vi "GUI - WaveFile (V2.00).vi"(0 "Time Data IN":refnum<class "GSwFormDSP.lvclass">, 5 "error in (no error)":errorcluster, 6 "Scale Factor":dbl=1.0 min=0.999993656453662 format="%#.2g", 7 "Application Name":string="GSwForm", 8 "Filename Option (Write)":T2(ring), 9 "State Queue":string[](array[string])=["SC >>> Initialize"], 11 "Wave - READ":path, 13 "Wave - WRITE":path) -> (14 "SubVI Time Data DUP":refnum<class "GSwFormDSP.lvclass">, 19 "error out":errorcluster)   [LabVIEW 2022 SP3, in "WaveFile.lvclass"]
uses:
  WaveFile.lvclass
  API/GSwFormDSP_class/GSwFormDSP.lvclass
  protected/Multi Signals Save Option.ctl
  <vilib>/Utility/sysdir.llb/System Directory Type.ctl
  W:/projects/archives/23 Charette AI Group/SPWB/API/Generic Utilities_class/Generic Utilities.lvclass
  API/Generic Utilities_class/Generic Utilities.lvclass
  <vilib>/addons/_AddQ/G#Object/G#Object.lvclass
panel:
  in  "Task":T1(tab)
  in  "READ - Multiple Files":path[](array[path])
  out "Time Data - READ":waveform(dbl)[](graph)
  in  "READ - Select Wave File":bool
  in  "READ - Select Multiple Wave File":bool
  in  "Multi Signal Save Option":T3
  out "Signal Name Tag":string="{ Signal Name }"
  in  "Open New TDF window":bool caption="Open the new Wave File in a New TDF window"
  in  "Suffix":string
  in  "Extension":string=".wav"
  in  "Fade IN and OUT":bool
  in  "Force Fs=44100Hz":bool
  in  "Filename":string
  in  "Unit Option":enum16{"No Change", "dB (Ref 20e-6 EU)"}(ring)
  in  "Unit":string
  in  "Save (GUI)":bool
  out "State History":string[](array[string])
  out "State Index":i32
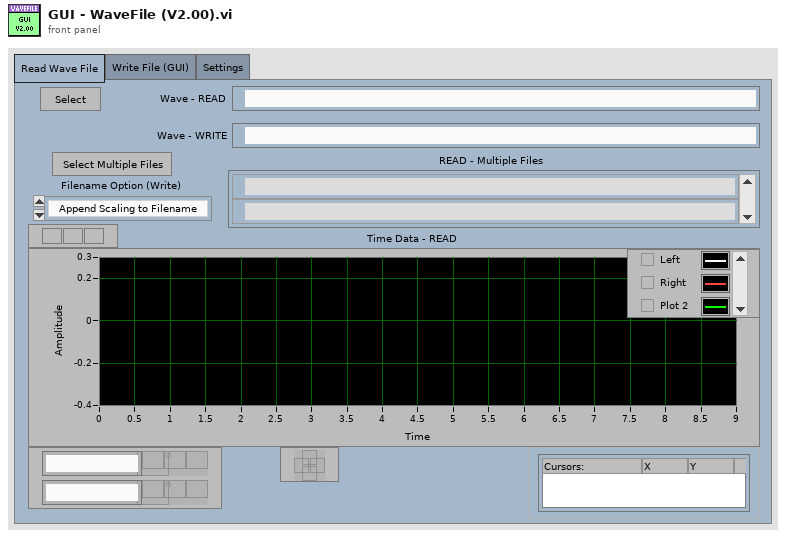
[diagram p1: front panel]
types:
  T1 = enum32{"Read Wave File", "Write File (GUI)", "Settings"}
  T2 = enum16{"Append Scaling to Filename", "No Scaling Info"}
  T3 = typedef "WaveFile.lvclass/Multi Signals Save Option.ctl" = enum16{"One wave file per signal", "Concatenate ALL signals to a single file", "Stereo (Ch1 is Left, Ch2 is Right)", "Stereo (Ch1 is Right, Ch2 is Left)"}
  T4 = enum8{"Enabled", "Disabled", "Disabled and Grayed Out"}
  T5 = enum32{"Invalid", "Standard", "Closed", "Hidden", "Minimized", "Maximized"}
  T6 = enum32{"Invalid", "Default", "Floating", "Floating/Auto-Hide", "Modal"}
  T7 = typedef "System Directory Type.ctl" = i32
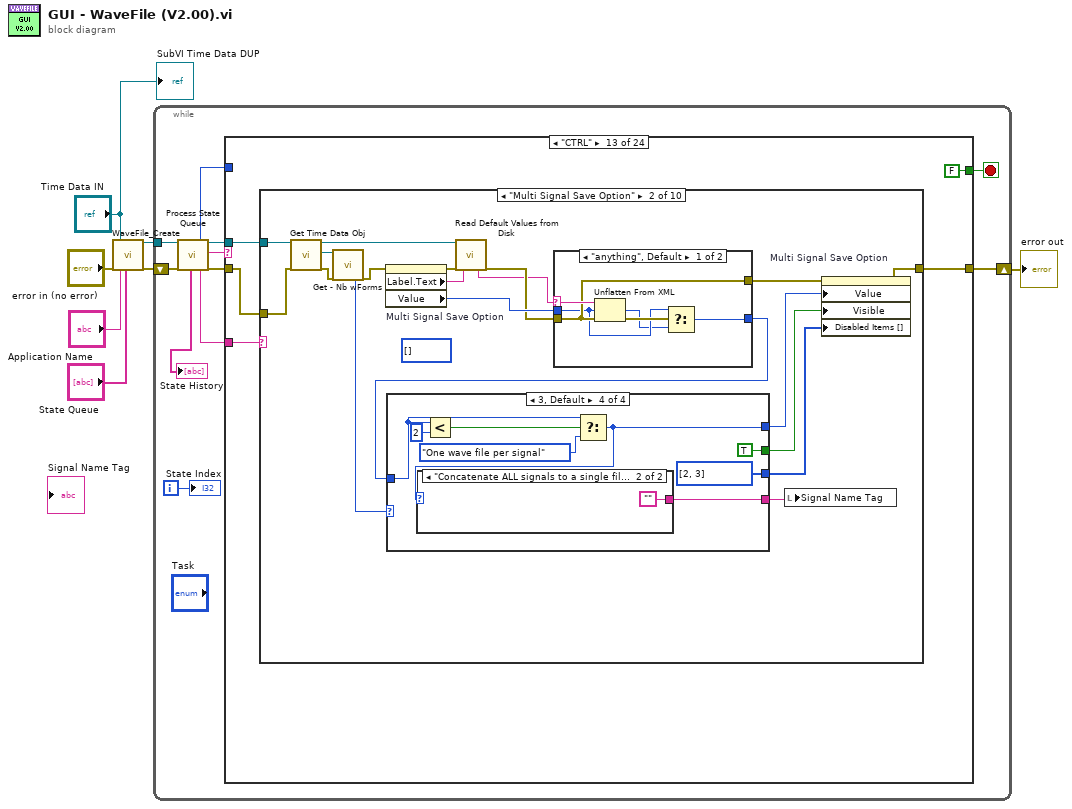
[diagram p0: block diagram]
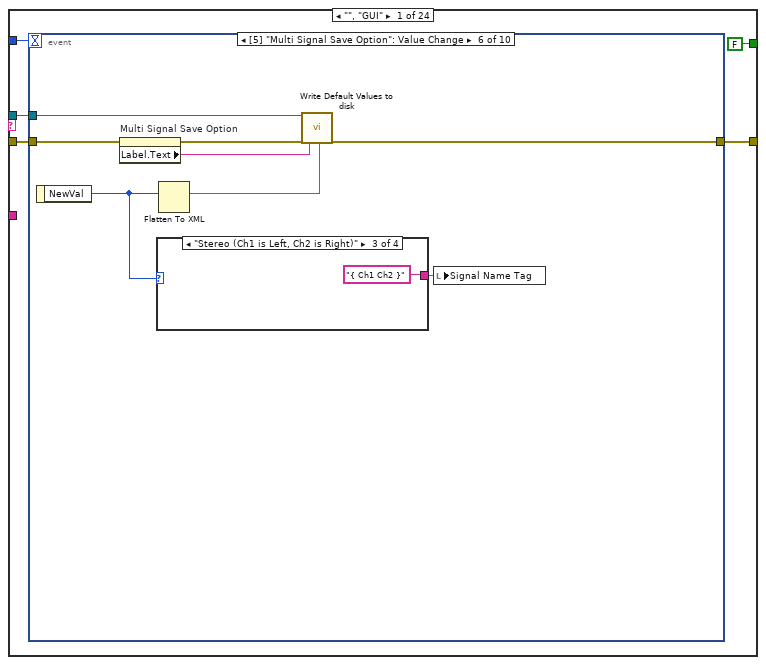
[diagram p2: hidden frame]
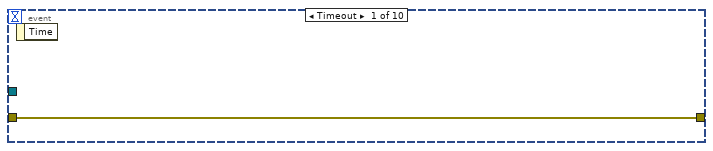
[diagram p3: hidden frame]
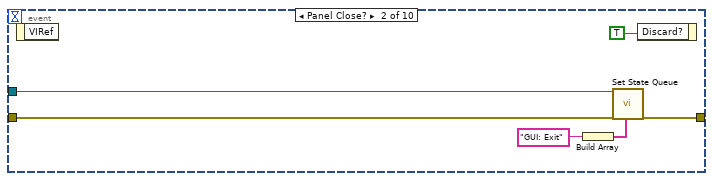
[diagram p4: hidden frame]
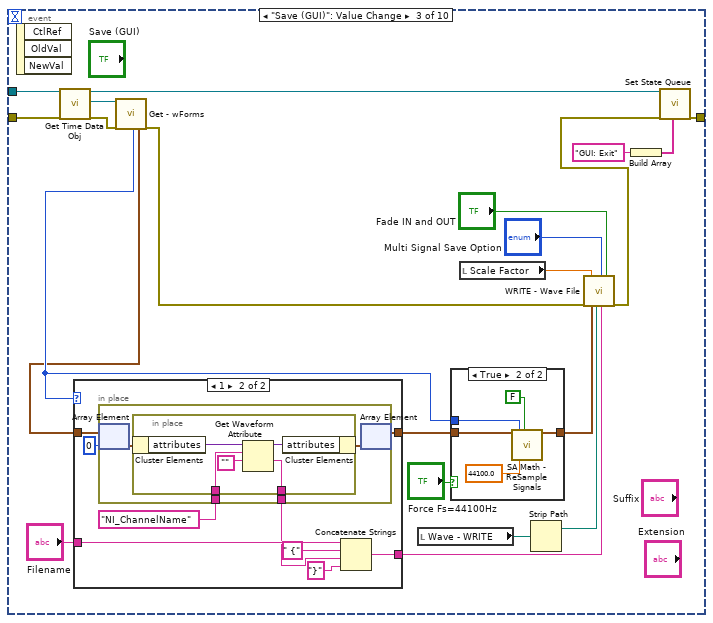
[diagram p5: hidden frame]
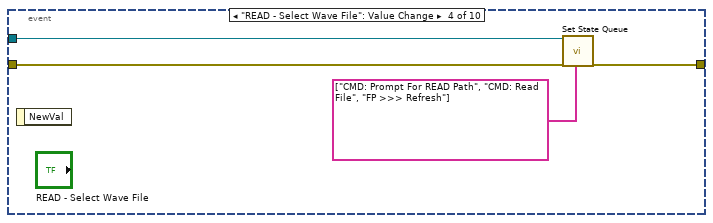
[diagram p8: hidden frame]
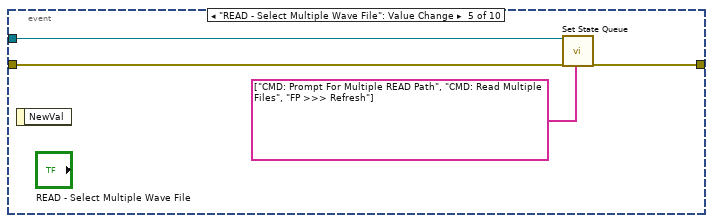
[diagram p9: hidden frame]
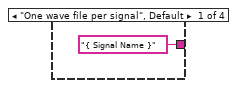
[diagram p10: hidden frame]
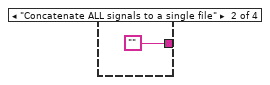
[diagram p11: hidden frame]
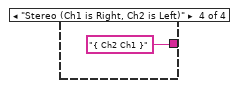
[diagram p12: hidden frame]
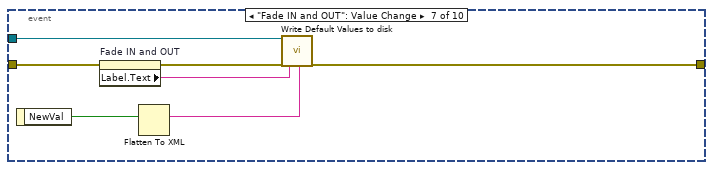
[diagram p13: hidden frame]
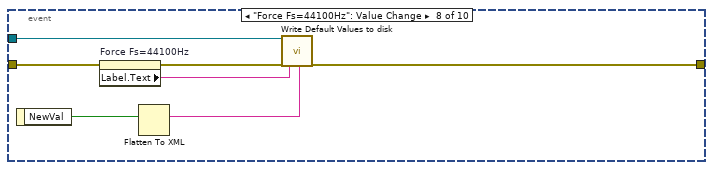
[diagram p14: hidden frame]
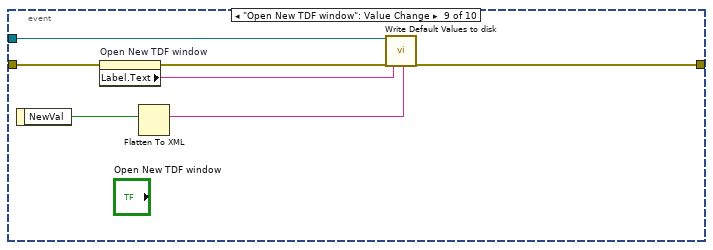
[diagram p15: hidden frame]
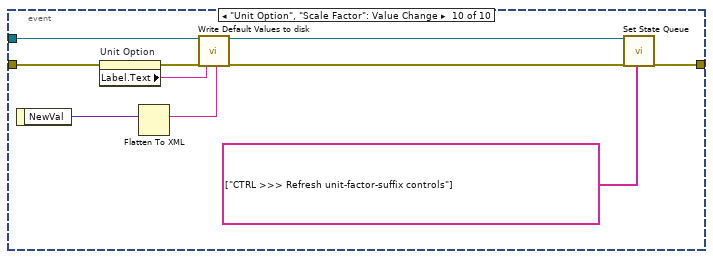
[diagram p16: hidden frame]
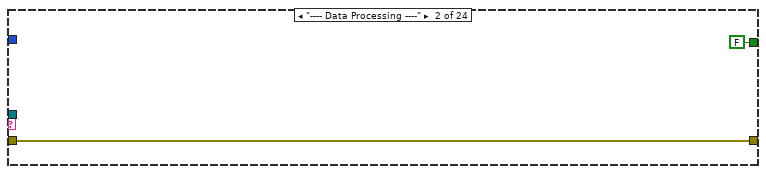
[diagram p17: hidden frame]
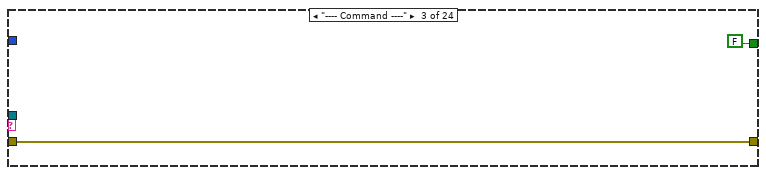
[diagram p18: hidden frame]
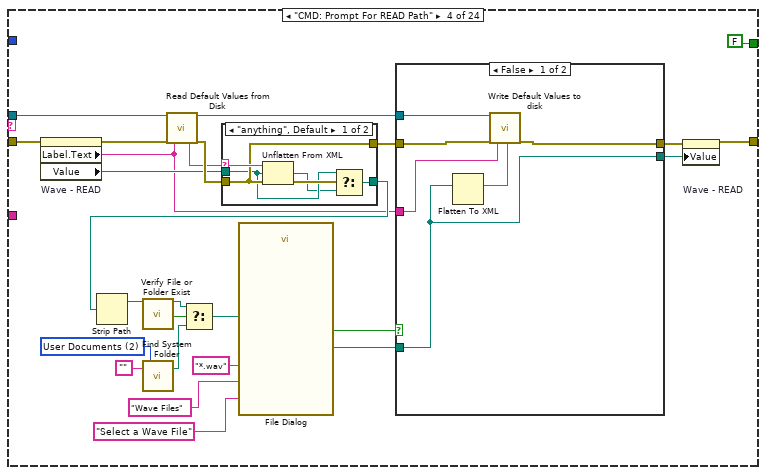
[diagram p19: hidden frame]
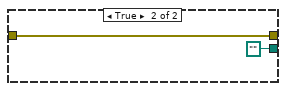
[diagram p20: hidden frame]
diagram:
  n1 = call "WaveFile_Create.vi"("error in (no error)"="error in (no error)", "Time Data"="Time Data IN", "Application Name"="Application Name", "State Queue"="State Queue") -> ("reference out"=w7:refnum<class "WaveFile.lvclass">, "error out"=w6:errorcluster)  [unwired: 14 in]
  n2 = while {
    shift-right: [w9] -> w2
    shift-left: w6 -> [w15]
    tunnel: w7 -> [w16]
    i -> [w17]
    stop <- w18 stop-if-true
    n3 = call "Process State Queue.vi"("reference in"=w16, "error in (no error)"=w15) -> ("State History"=→"State History":string[], "Timeout"=w14:i32, "State Option"=w11:string, "reference out"=w13:refnum<class "WaveFile.lvclass">, "Current State"=w12:string, "error out"=w10:errorcluster)  [unwired: 10 in, 2 out]
    n4 = case shown="\"CTRL\"" w12 {
      selector: w12 -> [_ _ _ _ _ _ _ _ _ _ _ _ _ _ _ _ _ _ _ _ w668 _ _ _]
      tunnel: w13 -> [w21 _ _ w158 w201 w243 w269 w280 w288 _ w316 _ w324 w530 _ w571 w594 w625 w650 _ _ _ _ w677]
      tunnel: [FALSE FALSE FALSE FALSE FALSE FALSE FALSE FALSE FALSE FALSE FALSE FALSE FALSE FALSE FALSE FALSE TRUE FALSE FALSE FALSE FALSE FALSE FALSE TRUE] -> w18
      tunnel: w14 -> [w22 _ _ _ _ _ _ _ _ _ _ _ _ _ _ _ _ _ _ _ _ _ _ _]
      tunnel: w11 -> [_ _ _ _ _ _ _ _ _ _ w312 _ w325 w527 _ w564 _ w634 _ _ _ _ _ _]
      tunnel: w10 -> [w20 w130 w132 w157 w200 w242 w268 w279 w290 w310 w315 w320 w322 w529 w554 w568 w591 w624 w651 w664 w666 w671 w674 w676]
      tunnel: [w19 w130 w132 w141 w185 w226 w267 w278 w289 w310 w314 w320 w323 w528 w554 w556 w590 w622 w647 w664 w666 errorcluster {"status"=FALSE, "code"=0, "source"=""} ("error out") w674 w678] -> w9
      frame "", "GUI" {
        n5 = event shown="[5] \"Multi Signal Save Option\": Value Change" {
          selector: _ -> [_ _ _ _ _ _ _ _ _ _]
          dyn-events: _ -> [_ _ _ _ _ _ _ _ _ _]
          timeout: w22 -> [_ _ _ _ _ _ _ _ _ _]
          tunnel: w21 -> [_ w28 w49 w81 w85 w93 w104 w111 w118 w128]
          tunnel: w20 -> [w24 w27 w48 w80 w84 w94 w105 w112 w119 w129]
          tunnel: [w24 w26 w50 w82 w86 w89 w99 w106 w113 w121] -> w19
          event Timeout {
            n6 = event-data() -> ()  [unwired: 1 in, 1 out]
          }
          event Panel Close? {
            n7 = event-data() -> ()  [unwired: 1 in, 1 out]
            n8 = Build Array("GUI: Exit") -> (w25:string[])
            n9 = call "Set State Queue.vi"("reference in"=w28, "error in (no error)"=w27, "State Queue"=w25) -> ("error out"=w26:errorcluster)  [unwired: 15 in, 1 out]
            n10 = event-data("Discard?"=TRUE) -> ()  [unwired: 1 in, 1 out]
          }
          event "Save (GUI)": Value Change {
            n11 = event-data() -> ()  [unwired: 1 in, 3 out]
            n12 = call "Get Time Data Obj.vi"("reference in"=w49, "error in (no error)"=w48) -> ("reference out"=w45:refnum<class "WaveFile.lvclass">, "Time data ref"=w47:refnum<class "GSwFormDSP.lvclass">, "error out"=w46:errorcluster)  [unwired: 15 in]
            n13 = call-dynamic "Get - wForms.vi"("reference in"=w47, "error in (no error)"=w46) -> ("Nb Signals"=w34:i32, "wForms"=w33:waveform(dbl)[], "error out"=w41:errorcluster)  [unwired: 14 in, 1 out]
            n14 = case shown="1" w34 {
              tunnel: [w54 w57] -> w38
              tunnel: "Filename" -> [w54 w60]
              tunnel: [w53 w62] -> w37
              tunnel: w33 -> [w53 w63]
              frame 0, Default {
              }
              frame 1 {
                n15 = in-place {
                  in-place-border: "NI_ChannelName" ("Att - wform Name") -> [w65]
                  in-place-border: [w64] -> w58
                  n16 = in-place-array #1(w63, 0) -> (w67:waveform(dbl))
                  n17 = in-place {
                    in-place-border: w65 -> [w70]
                    in-place-border: [w68] -> w64
                    n18 = in-place-cluster #2(w67) -> ("attributes"=w72:variant)
                    n19 = Get Waveform Attribute(5:"", 6:w70, 7:w72) -> (1:w68:string, 3:w71:variant)  [unwired: 1 in, 2 out]
                    n20 = in-place-cluster #2("attributes"=w71) -> (w66:waveform(dbl))
                  }
                  n21 = in-place-array #1(w66) -> (w62:waveform(dbl)[])  [unwired: 1 out]
                }
                n22 = Concatenate Strings(w60, " {" ("string"), w58, "}" ("string")) -> (w57:string)
              }
            }
            n23 = local read "Wave - WRITE"() -> (w42:path)
            n24 = case shown="True" "Force Fs=44100Hz" {
              tunnel: [w73 w77] -> w43
              tunnel: w37 -> [w73 w78]
              tunnel: w34 -> [_ w74]
              frame False {
              }
              frame True {
                n25 = call "SA Math - ReSample Signals.vi"("Time in"=w78, "Nb Signals"=w74, "New Fs"=44100.0, "Anotate Signal Name"=FALSE) -> ("Time out"=w77:waveform(dbl)[])  [unwired: 14 in, 1 out]
              }
            }
            n26 = local read "Scale Factor"() -> (w35:dbl)
            n27 = Strip Path(path=w42) -> (stripped path=w40:path)  [unwired: 1 out]
            n28 = call "WRITE - Wave File.vi"("error in (no error)"=w41, "Scaling Factor"=w35, "wForms"=w43, "Path"=w40, "Multi Signal Save Option"="Multi Signal Save Option", "Filename"=w38, "Fade IN and OUT"="Fade IN and OUT") -> ("error out"=w36:errorcluster)  [unwired: 12 in]
            n29 = Build Array("GUI: Exit") -> (w51:string[])
            n30 = call "Set State Queue.vi"("reference in"=w45, "error in (no error)"=w36, "State Queue"=w51) -> ("error out"=w50:errorcluster)  [unwired: 15 in, 1 out]
          }
          event "READ - Select Wave File": Value Change {
            n31 = event-data() -> ()  [unwired: 1 in, 1 out]
            n32 = call "Set State Queue.vi"("reference in"=w81, "error in (no error)"=w80, "State Queue"=string[] ["CMD: Prompt For READ Path", "CMD: Read File", "FP >>> Refresh"]) -> ("error out"=w82:errorcluster)  [unwired: 15 in, 1 out]
          }
          event "READ - Select Multiple Wave File": Value Change {
            n33 = event-data() -> ()  [unwired: 1 in, 1 out]
            n34 = call "Set State Queue.vi"("reference in"=w85, "error in (no error)"=w84, "State Queue"=string[] ["CMD: Prompt For Multiple READ Path", "CMD: Read Multiple Files", "FP >>> Refresh"]) -> ("error out"=w86:errorcluster)  [unwired: 15 in, 1 out]
          }
          event Value Change {
            n35 = event-data() -> ("NewVal"=w88:T3)  [unwired: 1 in]
            n36 = property on="Multi Signal Save Option" class="Enum (strict)"(error in=w94) -> (error out=w92:errorcluster, "Label.Text"=w91:string)  [unwired: 1 in, 1 out]
            n37 = case shown="\"Stereo (Ch1 is Left, Ch2 is Right)\"" w88 {
              tunnel: ["{ Signal Name }" "" "{ Ch1 Ch2 }" "{ Ch2 Ch1 }"] -> w87
              frame "One wave file per signal", Default {
              }
              frame "Concatenate ALL signals to a single file" {
              }
              frame "Stereo (Ch1 is Left, Ch2 is Right)" {
              }
              frame "Stereo (Ch1 is Right, Ch2 is Left)" {
              }
            }
            n38 = Flatten To XML(6:w88) -> (2:w90:string)
            n39 = call-dynamic "Write Default Values to disk.vi"("reference in"=w93, "error in (no error)"=w92, "Control Label"=w91, "Value (XML String)"=w90) -> ("error out"=w89:errorcluster)  [unwired: 14 in, 1 out]
            n40 = local write "Signal Name Tag"(w87) -> ()
          }
          event "Fade IN and OUT": Value Change {
            n41 = event-data() -> ("NewVal"=w101:bool)  [unwired: 1 in]
            n42 = property on="Fade IN and OUT" class="Bool (strict)"(error in=w105) -> (error out=w103:errorcluster, "Label.Text"=w102:string)  [unwired: 1 in, 1 out]
            n43 = Flatten To XML(6:w101) -> (2:w100:string)
            n44 = call-dynamic "Write Default Values to disk.vi"("reference in"=w104, "error in (no error)"=w103, "Control Label"=w102, "Value (XML String)"=w100) -> ("error out"=w99:errorcluster)  [unwired: 14 in, 1 out]
          }
          event "Force Fs=44100Hz": Value Change {
            n45 = event-data() -> ("NewVal"=w108:bool)  [unwired: 1 in]
            n46 = property on="Force Fs=44100Hz" class="Bool (strict)"(error in=w112) -> (error out=w110:errorcluster, "Label.Text"=w109:string)  [unwired: 1 in, 1 out]
            n47 = Flatten To XML(6:w108) -> (2:w107:string)
            n48 = call-dynamic "Write Default Values to disk.vi"("reference in"=w111, "error in (no error)"=w110, "Control Label"=w109, "Value (XML String)"=w107) -> ("error out"=w106:errorcluster)  [unwired: 14 in, 1 out]
          }
          event "Open New TDF window": Value Change {
            n49 = event-data() -> ("NewVal"=w115:bool)  [unwired: 1 in]
            n50 = property on="Open New TDF window" class="Bool (strict)"(error in=w119) -> (error out=w117:errorcluster, "Label.Text"=w116:string)  [unwired: 1 in, 1 out]
            n51 = Flatten To XML(6:w115) -> (2:w114:string)
            n52 = call-dynamic "Write Default Values to disk.vi"("reference in"=w118, "error in (no error)"=w117, "Control Label"=w116, "Value (XML String)"=w114) -> ("error out"=w113:errorcluster)  [unwired: 14 in, 1 out]
          }
          event "Unit Option", "Scale Factor": Value Change {
            n53 = event-data() -> ("NewVal"=w125:variant)  [unwired: 1 in]
            n54 = property on="Unit Option" class="Enum (strict)"(error in=w129) -> (error out=w127:errorcluster, "Label.Text"=w126:string)  [unwired: 1 in, 1 out]
            n55 = Flatten To XML(6:w125) -> (2:w124:string)
            n56 = call-dynamic "Write Default Values to disk.vi"("reference in"=w128, "error in (no error)"=w127, "Control Label"=w126, "Value (XML String)"=w124) -> ("reference out"=w120:refnum<class "WaveFile.lvclass">, "error out"=w122:errorcluster)  [unwired: 14 in]
            n57 = call "Set State Queue.vi"("reference in"=w120, "error in (no error)"=w122, "State Queue"=string[] ["CTRL >>> Refresh unit-factor-suffix controls"]) -> ("error out"=w121:errorcluster)  [unwired: 15 in, 1 out]
          }
        }
      }
      frame "---- Data Processing ----" {
      }
      frame "---- Command ----" {
      }
      frame "CMD: Prompt For READ Path" {
        w148 = T7 2 items=["User Home"=0, "User Desktop"=1, "User Documents"=2, "User Application Data"=3, "User Preferences"=4, "User Temporary"=5, "Public Documents"=6, "Public Application Data"=7, "Public Preferences"=8, "Public Cache"=13, "System Core Libraries"=9, "System Installed Libraries"=10, "Application Files"=11, "Boot Volume Root"=12] ("system directory type")
        n58 = property on="Wave - READ" class="Path"(error in=w157) -> (error out=w156:errorcluster, "Label.Text"=w136:string, "Value"=w154:path)  [unwired: 1 in, 1 out]
        n59 = call "Find System Folder.vi"("Application Name"="", "system directory type"=w148) -> ("System Folder"=w147:path)  [unwired: 16 in, 1 out]
        n60 = call-dynamic "Read Default Values from Disk.vi"("reference in"=w158, "error in (no error)"=w156, "Control Label"=w136) -> ("Value (XML String)"=w134:string, "reference out"=w137:refnum<class "WaveFile.lvclass">, "error out"=w155:errorcluster)  [unwired: 14 in]
        n61 = case shown="\"anything\", Default" w134 {
          selector: w134 -> [w173 _]
          tunnel: [w168 w175] -> w153
          tunnel: w154 -> [w170 w175]
          tunnel: w155 -> [w171 w174]
          tunnel: [w171 w174] -> w139
          frame "anything", Default {
            n62 = Unflatten From XML(xml string=w173, type=w170, error in (no error)=w171) -> (value=w169:path, error out=w172:errorcluster)
            n63 = Select(t=w170, s=w172, f=w169) -> (s? t:f=w168:path)
          }
          frame "" {
            # "Either the file was not found or there was some error"
          }
        }
        n64 = Strip Path(path=w153) -> (stripped path=w152:path)  [unwired: 1 out]
        n65 = call "Verify File or Folder Exist.vi"("path"=w152) -> ("dup path"=w150:path, "file or folder exists?"=w151:bool)  [unwired: 16 in, 1 out]
        n66 = Select(t=w150, s=w151, f=w147) -> (s? t:f=w149:path)
        n67 = call "File Dialog"("start path"=w149, "button label"="Select a Wave File", "pattern (all files)"="*.wav", "pattern label"="Wave Files") -> ("selected path"=w135:path, "cancelled"=w142:bool)  [unwired: 8 in, 2 out]
        n68 = case shown="False" w142 {
          tunnel: [w161 w167] -> w140
          tunnel: w139 -> [w162 w167]
          tunnel: [w160 path ""] -> w138
          tunnel: w137 -> [w164 _]
          tunnel: w136 -> [w163 _]
          tunnel: w135 -> [w160 _]
          frame False {
            n69 = Flatten To XML(6:w160) -> (2:w165:string)
            n70 = call-dynamic "Write Default Values to disk.vi"("reference in"=w164, "error in (no error)"=w162, "Control Label"=w163, "Value (XML String)"=w165) -> ("error out"=w161:errorcluster)  [unwired: 14 in, 1 out]
          }
          frame True {
          }
        }
        n71 = property on="Wave - READ" class="Path"(error in=w140, "Value"=w138) -> (error out=w141:errorcluster)  [unwired: 1 in, 1 out]
      }
      frame "CMD: Prompt For Multiple READ Path" {
        w192 = T7 2 items=["User Home"=0, "User Desktop"=1, "User Documents"=2, "User Application Data"=3, "User Preferences"=4, "User Temporary"=5, "Public Documents"=6, "Public Application Data"=7, "Public Preferences"=8, "Public Cache"=13, "System Core Libraries"=9, "System Installed Libraries"=10, "Application Files"=11, "Boot Volume Root"=12] ("system directory type")
        n72 = property on="READ - Multiple Files" class="Arr (strict)"(error in=w200) -> (error out=w199:errorcluster, "Label.Text"=w180:string, "Value"=w197:path[])  [unwired: 1 in, 1 out]
        n73 = call "Find System Folder.vi"("Application Name"="", "system directory type"=w192) -> ("System Folder"=w191:path)  [unwired: 16 in, 1 out]
        n74 = call-dynamic "Read Default Values from Disk.vi"("reference in"=w201, "error in (no error)"=w199, "Control Label"=w180) -> ("Value (XML String)"=w176:string, "reference out"=w181:refnum<class "WaveFile.lvclass">, "error out"=w198:errorcluster)  [unwired: 14 in]
        n75 = case shown="\"anything\", Default" w176 {
          selector: w176 -> [w216 _]
          tunnel: [w211 w218] -> w179
          tunnel: w197 -> [w213 w218]
          tunnel: w198 -> [w214 w217]
          tunnel: [w214 w217] -> w183
          frame "anything", Default {
            n76 = Unflatten From XML(xml string=w216, type=w213, error in (no error)=w214) -> (value=w212:path[], error out=w215:errorcluster)
            n77 = Select(t=w213, s=w215, f=w212) -> (s? t:f=w211:path[])
          }
          frame "" {
            # "Either the file was not found or there was some error"
          }
        }
        n78 = Index Array(array=w179) -> (element=w178:path)  [unwired: 1 in]
        n79 = Strip Path(path=w178) -> (stripped path=w196:path)  [unwired: 1 out]
        n80 = call "Verify File or Folder Exist.vi"("path"=w196) -> ("dup path"=w194:path, "file or folder exists?"=w195:bool)  [unwired: 16 in, 1 out]
        n81 = Select(t=w194, s=w195, f=w191) -> (s? t:f=w193:path)
        n82 = call "Multi Wave Files"("start path"=w193, "button label"="Select One or More Wave Files", "pattern (all files)"="*.wav", "pattern label"="Wave Files") -> ("selected paths"=w177:path[], "cancelled"=w186:bool)  [unwired: 8 in, 2 out]
        n83 = case shown="False" w186 {
          tunnel: [w204 w210] -> w184
          tunnel: w183 -> [w205 w210]
          tunnel: [w203 path[] [] ("selected paths")] -> w182
          tunnel: w181 -> [w207 _]
          tunnel: w180 -> [w206 _]
          tunnel: w177 -> [w203 _]
          frame False {
            n84 = Flatten To XML(6:w203) -> (2:w208:string)
            n85 = call-dynamic "Write Default Values to disk.vi"("reference in"=w207, "error in (no error)"=w205, "Control Label"=w206, "Value (XML String)"=w208) -> ("error out"=w204:errorcluster)  [unwired: 14 in, 1 out]
          }
          frame True {
          }
        }
        n86 = property on="READ - Multiple Files" class="Arr (strict)"(error in=w184, "Value"=w182) -> (error out=w185:errorcluster)  [unwired: 1 in, 1 out]
      }
      frame "CMD: Prompt For WRITE Path" {
        w233 = T7 2 items=["User Home"=0, "User Desktop"=1, "User Documents"=2, "User Application Data"=3, "User Preferences"=4, "User Temporary"=5, "Public Documents"=6, "Public Application Data"=7, "Public Preferences"=8, "Public Cache"=13, "System Core Libraries"=9, "System Installed Libraries"=10, "Application Files"=11, "Boot Volume Root"=12] ("system directory type")
        n87 = property on="Wave - WRITE" class="Path"(error in=w242) -> (error out=w241:errorcluster, "Label.Text"=w221:string, "Value"=w239:path)  [unwired: 1 in, 1 out]
        n88 = call "Find System Folder.vi"("Application Name"="", "system directory type"=w233) -> ("System Folder"=w232:path)  [unwired: 16 in, 1 out]
        n89 = call-dynamic "Read Default Values from Disk.vi"("reference in"=w243, "error in (no error)"=w241, "Control Label"=w221) -> ("Value (XML String)"=w219:string, "reference out"=w222:refnum<class "WaveFile.lvclass">, "error out"=w240:errorcluster)  [unwired: 14 in]
        n90 = case shown="\"anything\", Default" w219 {
          selector: w219 -> [w262 _]
          tunnel: [w257 w264] -> w238
          tunnel: w239 -> [w259 w264]
          tunnel: w240 -> [w260 w263]
          tunnel: [w260 w263] -> w224
          frame "anything", Default {
            n91 = Unflatten From XML(xml string=w262, type=w259, error in (no error)=w260) -> (value=w258:path, error out=w261:errorcluster)
            n92 = Select(t=w259, s=w261, f=w258) -> (s? t:f=w257:path)
          }
          frame "" {
            # "Either the file was not found or there was some error"
          }
        }
        n93 = Strip Path(path=w238) -> (stripped path=w237:path)  [unwired: 1 out]
        n94 = call "Verify File or Folder Exist.vi"("path"=w237) -> ("dup path"=w235:path, "file or folder exists?"=w236:bool)  [unwired: 16 in, 1 out]
        n95 = Select(t=w235, s=w236, f=w232) -> (s? t:f=w234:path)
        n96 = call "File Write"("start path"=w234, "button label"="Select a Wave File", "pattern (all files)"="*.wav", "pattern label"="Wave Files") -> ("selected path"=w220:path, "cancelled"=w227:bool)  [unwired: 8 in, 2 out]
        n97 = case shown="False" w227 {
          tunnel: [w246 w251] -> w225
          tunnel: w224 -> [w247 w252]
          tunnel: [w245 path ""] -> w223
          tunnel: w222 -> [w249 w253]
          tunnel: w221 -> [w248 _]
          tunnel: w220 -> [w245 _]
          frame False {
            n98 = Flatten To XML(6:w245) -> (2:w250:string)
            n99 = call-dynamic "Write Default Values to disk.vi"("reference in"=w249, "error in (no error)"=w247, "Control Label"=w248, "Value (XML String)"=w250) -> ("error out"=w246:errorcluster)  [unwired: 14 in, 1 out]
          }
          frame True {
            n100 = Build Array("Quit") -> (w254:string[])
            n101 = call "Set State Queue.vi"("reference in"=w253, "error in (no error)"=w252, "State Queue"=w254) -> ("error out"=w251:errorcluster)  [unwired: 15 in, 1 out]
          }
        }
        n102 = property on="Wave - WRITE" class="Path"(error in=w225, "Value"=w223) -> (error out=w226:errorcluster)  [unwired: 1 in, 1 out]
      }
      frame "CMD: Read File" {
        n103 = Empty String/Path?(string/path="Wave - READ") -> (empty?=w265:bool)
        n104 = case shown="False" w265 {
          tunnel: w269 -> [w274 _]
          tunnel: w268 -> [w273 w275]
          tunnel: [w271 w275] -> w267
          tunnel: "Wave - READ" -> [w272 _]
          frame False {
            n105 = call "READ - Wave File.vi"("reference in"=w274, "error in (no error)"=w273, "Wave File Path - READ"=w272) -> ("error out"=w271:errorcluster)  [unwired: 15 in, 1 out]
          }
          frame True {
            # "User cancelled, so do nothing!"
          }
        }
      }
      frame "CMD: Read Multiple Files" {
        n106 = Empty Array?(array="READ - Multiple Files") -> (empty?=w277:bool)
        n107 = case shown="False" w277 {
          tunnel: w280 -> [w285 _]
          tunnel: w279 -> [w284 w286]
          tunnel: [w282 w286] -> w278
          tunnel: "READ - Multiple Files" -> [w283 _]
          frame False {
            n108 = call "READ - Multiple Wave Files.vi"("reference in"=w285, "error in (no error)"=w284, "READ - Multiple Files"=w283) -> ("error out"=w282:errorcluster)  [unwired: 15 in, 1 out]
          }
          frame True {
            # "User cancelled, so do nothing!"
          }
        }
      }
      frame "CMD: Write File" {
        n109 = Empty String/Path?(string/path="Wave - WRITE") -> (empty?=w291:bool)
        n110 = case shown="False" w291 {
          tunnel: w290 -> [w306 w309]
          tunnel: [w308 w309] -> w289
          tunnel: w288 -> [w307 _]
          tunnel: "Wave - WRITE" -> [w302 _]
          frame False {
            (unwired) ""
            n111 = call "Get Time Data Obj.vi"("reference in"=w307, "error in (no error)"=w306) -> ("Time data ref"=w295:refnum<class "GSwFormDSP.lvclass">, "error out"=w296:errorcluster)  [unwired: 15 in, 1 out]
            n112 = call <vilib>:"Get File Extension.vi"("file"=w302) -> ("filename without extension"=w300:string, "dup file"=w301:path)  [unwired: 6 in, 3 out]
            n113 = call-dynamic "Conditionning - Taper wForms.vi"("reference in"=w295, "error in (no error)"=w296, "Anotate Signal Name"=FALSE) -> ("reference in"=w298:refnum<class "GSwFormDSP.lvclass">, "error out"=w297:errorcluster)  [unwired: 15 in]
            n114 = Strip Path(path=w301) -> (stripped path=w303:path)  [unwired: 1 out]
            n115 = local read "Scale Factor"() -> (w299:dbl)
            n116 = call-dynamic "Get - wForms.vi"("reference in"=w298, "error in (no error)"=w297) -> ("wForms"=w304:waveform(dbl)[], "error out"=w305:errorcluster)  [unwired: 14 in, 2 out]
            n117 = call "WRITE - Wave File.vi"("error in (no error)"=w305, "Scaling Factor"=w299, "wForms"=w304, "Filename Option"="Filename Option (Write)", "Path"=w303, "Filename"=w300) -> ("error out"=w308:errorcluster)  [unwired: 13 in]
          }
          frame True {
            # "User cancelled, so do nothing!"
          }
        }
      }
      frame "---- Scripts ----" {
      }
      frame "SC" {
        n118 = case shown="\"Init GUI Write\"" w312 {
          tunnel: [string[] ["GUI: Initialize Ref", "FP >>> Open"] ("State Queue OUT") string[] ["GUI: Initialize Ref >>> GUI Write", "CTRL >>> Unit Option", "CTRL >>> GUI Write - Task Tab", "CTRL >>> GUI Write - Filename", "CTRL >>> GUI Write - Scale Factor and Unit", "CTRL >>> Multi Signal Save Option", "CTRL >>> Fade IN and OUT", "CTRL >>> Fs = 44100Hz", "CTRL >>> Refresh unit-factor-suffix controls", "CTRL >>> Open New TDF Window", "FP >>> Open"] ("State Queue OUT")] -> w313
          frame "Initialize", Default {
          }
          frame "Init GUI Write" {
          }
        }
        n119 = call "Set State Queue.vi"("reference in"=w316, "error in (no error)"=w315, "State Queue"=w313) -> ("error out"=w314:errorcluster)  [unwired: 15 in, 1 out]
      }
      frame "---- Front Panel Mgmt ----" {
      }
      frame "CTRL" {
        n120 = case shown="\"Multi Signal Save Option\"" w325 {
          selector: w325 -> [w329 _ _ _ _ _ _ _ _ _]
          tunnel: w324 -> [_ w342 w391 w409 w427 w445 _ _ w492 _]
          tunnel: [w327 w344 w386 w404 w422 w440 w456 w470 w480 w495] -> w323
          tunnel: w322 -> [w327 w343 w389 w407 w425 w443 w459 w473 w491 w493]
          frame "unknown", Default {
            n121 = Concatenate Strings("The following control name is unrecognized:\n", w329) -> (w328:string)
            n122 = One Button Dialog(message=w328) -> ()  [unwired: 1 in, 1 out]
          }
          frame "Multi Signal Save Option" {
            (unwired) i32[] [] ("Disabled Items []")
            n123 = call "Get Time Data Obj.vi"("reference in"=w342, "error in (no error)"=w343) -> ("reference out"=w336:refnum<class "WaveFile.lvclass">, "Time data ref"=w341:refnum<class "GSwFormDSP.lvclass">, "error out"=w340:errorcluster)  [unwired: 15 in]
            n124 = call-dynamic "Get - Nb wForms.vi"("reference in"=w341, "error in (no error)"=w340) -> ("Nb Wave Forms"=w334:i32, "error out"=w339:errorcluster)  [unwired: 15 in, 1 out]
            n125 = property on="Multi Signal Save Option" class="Enum (strict)"(error in=w339) -> (error out=w347:errorcluster, "Label.Text"=w346:string, "Value"=w349:T3)  [unwired: 1 in, 1 out]
            n126 = call-dynamic "Read Default Values from Disk.vi"("reference in"=w336, "error in (no error)"=w347, "Control Label"=w346) -> ("Value (XML String)"=w335:string, "error out"=w345:errorcluster)  [unwired: 14 in, 1 out]
            n127 = case shown="\"anything\", Default" w335 {
              selector: w335 -> [w381 _]
              tunnel: [w376 w383] -> w338
              tunnel: w349 -> [w378 w383]
              tunnel: w345 -> [w379 w382]
              tunnel: [w379 w382] -> w348
              frame "anything", Default {
                n128 = Unflatten From XML(xml string=w381, type=w378, error in (no error)=w379) -> (value=w377:T3, error out=w380:errorcluster)
                n129 = Select(t=w378, s=w380, f=w377) -> (s? t:f=w376:T3)
              }
              frame "" {
                # "Either the file was not found or there was some error"
              }
            }
            n130 = case shown="3, Default" w334 {
              tunnel: w338 -> [_ _ w360 w369]
              tunnel: ["" "" w361 w370] -> w337
              tunnel: [Multi_Signals_Save_Option."One wave file per signal" ("Multi Signal Save Option") Multi_Signals_Save_Option."One wave file per signal" ("Multi Signal Save Option") w360 w366] -> w333
              tunnel: [FALSE FALSE TRUE TRUE] -> w332
              tunnel: [i32[] [0, 1, 2, 3] ("Disabled Items []") i32[] [1, 2, 3] ("Disabled Items []") i32[] [] ("Disabled Items []") i32[] [2, 3] ("Disabled Items []")] -> w331
              frame 0 {
              }
              frame 1 {
              }
              frame 2 {
                n131 = case shown="\"One wave file per signal\", Default" w360 {
                  tunnel: ["{ Signal Name }" "" "{ Ch1 Ch2 }" "{ Ch2 Ch1 }"] -> w361
                  frame "One wave file per signal", Default {
                  }
                  frame "Concatenate ALL signals to a single file" {
                    # "Create only 1 signal"
                  }
                  frame "Stereo (Ch1 is Left, Ch2 is Right)" {
                  }
                  frame "Stereo (Ch1 is Right, Ch2 is Left)" {
                  }
                }
              }
              frame 3, Default {
                n132 = Less?(x=w369, y=2) -> (x < y?=w373:bool)
                n133 = Select(t=w369, s=w373, f=Multi_Signals_Save_Option."One wave file per signal") -> (s? t:f=w366:T3)
                n134 = case shown="\"Concatenate ALL signals to a single file\"" w366 {
                  tunnel: ["{ Signal Name }" ""] -> w370
                  frame "One wave file per signal", Default {
                  }
                  frame "Concatenate ALL signals to a single file" {
                  }
                }
              }
            }
            n135 = local write "Signal Name Tag"(w337) -> ()
            n136 = property on="Multi Signal Save Option" class="Enum (strict)"(error in=w348, "Value"=w333, "Visible"=w332, "Disabled Items []"=w331) -> (error out=w344:errorcluster)  [unwired: 1 in, 1 out]
          }
          frame "Fade IN and OUT" {
            n137 = property on="Fade IN and OUT" class="Bool (strict)"(error in=w389) -> (error out=w390:errorcluster, "Label.Text"=w388:string, "Value"=w393:bool)  [unwired: 1 in, 1 out]
            n138 = call-dynamic "Read Default Values from Disk.vi"("reference in"=w391, "error in (no error)"=w390, "Control Label"=w388) -> ("Value (XML String)"=w384:string, "error out"=w387:errorcluster)  [unwired: 14 in, 1 out]
            n139 = case shown="\"anything\", Default" w384 {
              selector: w384 -> [w399 _]
              tunnel: [w394 w401] -> w385
              tunnel: w393 -> [w396 w401]
              tunnel: w387 -> [w397 w400]
              tunnel: [w397 w400] -> w392
              frame "anything", Default {
                n140 = Unflatten From XML(xml string=w399, type=w396, error in (no error)=w397) -> (value=w395:bool, error out=w398:errorcluster)
                n141 = Select(t=w396, s=w398, f=w395) -> (s? t:f=w394:bool)
              }
              frame "" {
                # "Either the file was not found or there was some error"
              }
            }
            n142 = property on="Fade IN and OUT" class="Bool (strict)"(error in=w392, "Value"=w385) -> (error out=w386:errorcluster)  [unwired: 1 in, 1 out]
          }
          frame "Fs = 44100Hz" {
            n143 = property on="Force Fs=44100Hz" class="Bool (strict)"(error in=w407) -> (error out=w408:errorcluster, "Label.Text"=w406:string, "Value"=w411:bool)  [unwired: 1 in, 1 out]
            n144 = call-dynamic "Read Default Values from Disk.vi"("reference in"=w409, "error in (no error)"=w408, "Control Label"=w406) -> ("Value (XML String)"=w402:string, "error out"=w405:errorcluster)  [unwired: 14 in, 1 out]
            n145 = case shown="\"anything\", Default" w402 {
              selector: w402 -> [w417 _]
              tunnel: [w412 w419] -> w403
              tunnel: w411 -> [w414 w419]
              tunnel: w405 -> [w415 w418]
              tunnel: [w415 w418] -> w410
              frame "anything", Default {
                n146 = Unflatten From XML(xml string=w417, type=w414, error in (no error)=w415) -> (value=w413:bool, error out=w416:errorcluster)
                n147 = Select(t=w414, s=w416, f=w413) -> (s? t:f=w412:bool)
              }
              frame "" {
                # "Either the file was not found or there was some error"
              }
            }
            n148 = property on="Force Fs=44100Hz" class="Bool (strict)"(error in=w410, "Value"=w403) -> (error out=w404:errorcluster)  [unwired: 1 in, 1 out]
          }
          frame "Open New TDF Window" {
            n149 = property on="Open New TDF window" class="Bool (strict)"(error in=w425) -> (error out=w426:errorcluster, "Label.Text"=w424:string, "Value"=w429:bool)  [unwired: 1 in, 1 out]
            n150 = call-dynamic "Read Default Values from Disk.vi"("reference in"=w427, "error in (no error)"=w426, "Control Label"=w424) -> ("Value (XML String)"=w420:string, "error out"=w423:errorcluster)  [unwired: 14 in, 1 out]
            n151 = case shown="\"anything\", Default" w420 {
              selector: w420 -> [w435 _]
              tunnel: [w430 w437] -> w421
              tunnel: w429 -> [w432 w437]
              tunnel: w423 -> [w433 w436]
              tunnel: [w433 w436] -> w428
              frame "anything", Default {
                n152 = Unflatten From XML(xml string=w435, type=w432, error in (no error)=w433) -> (value=w431:bool, error out=w434:errorcluster)
                n153 = Select(t=w432, s=w434, f=w431) -> (s? t:f=w430:bool)
              }
              frame "" {
                # "Either the file was not found or there was some error"
              }
            }
            n154 = property on="Open New TDF window" class="Bool (strict)"(error in=w428, "Value"=w421) -> (error out=w422:errorcluster)  [unwired: 1 in, 1 out]
          }
          frame "Unit Option" {
            n155 = property on="Unit Option" class="Enum (strict)"(error in=w443) -> (error out=w444:errorcluster, "Label.Text"=w442:string, "Value"=w447:enum16{"No Change", "dB (Ref 20e-6 EU)"})  [unwired: 1 in, 1 out]
            n156 = call-dynamic "Read Default Values from Disk.vi"("reference in"=w445, "error in (no error)"=w444, "Control Label"=w442) -> ("Value (XML String)"=w438:string, "error out"=w441:errorcluster)  [unwired: 14 in, 1 out]
            n157 = case shown="\"anything\", Default" w438 {
              selector: w438 -> [w453 _]
              tunnel: [w448 w455] -> w439
              tunnel: w447 -> [w450 w455]
              tunnel: w441 -> [w451 w454]
              tunnel: [w451 w454] -> w446
              frame "anything", Default {
                n158 = Unflatten From XML(xml string=w453, type=w450, error in (no error)=w451) -> (value=w449:enum16{"No Change", "dB (Ref 20e-6 EU)"}, error out=w452:errorcluster)
                n159 = Select(t=w450, s=w452, f=w449) -> (s? t:f=w448:enum16{"No Change", "dB (Ref 20e-6 EU)"})
              }
              frame "" {
                # "Either the file was not found or there was some error"
              }
            }
            n160 = property on="Unit Option" class="Enum (strict)"(error in=w446, "Value"=w439) -> (error out=w440:errorcluster)  [unwired: 1 in, 1 out]
          }
          frame "GUI Write - Task Tab" {
            n161 = property on="Task" class="TabCtl (strict)"(error in=w459, "Value"=T1."Write File (GUI)" ("Task"), "PageSelVis"=FALSE ("Page Selector Visible")) -> (error out=w456:errorcluster)  [unwired: 1 in, 1 out]
          }
          frame "GUI Write - Filename" {
            # "Remove any references"
            # "Remove any signal names"
            # "Remove extension if present!"
            n162 = property on="Wave - WRITE" class="Path"(error in=w473) -> (error out=w471:errorcluster, "Value"=w472:path)  [unwired: 1 in, 1 out]
            n163 = Strip Path(path=w472) -> (name=w465:string)  [unwired: 1 out]
            n164 = Reverse String(1:w465) -> (0:w469:string)
            n165 = Match Pattern(string=w469, regular expression="\\.") -> (after substring=w467:string, offset past match=w466:i32)  [unwired: 1 in, 2 out]
            n166 = case shown="0, Default" w466 {
              tunnel: w467 -> [w475 _]
              tunnel: [w474 w476] -> w461
              tunnel: w465 -> [_ w476]
              frame 0, Default {
                n167 = Reverse String(1:w475) -> (0:w474:string)
              }
              frame -1 {
              }
            }
            n168 = Match Pattern(string=w461, regular expression="{") -> (before substring=w460:string)  [unwired: 1 in, 3 out]
            n169 = Match Pattern(string=w460, regular expression="_scale") -> (before substring=w463:string)  [unwired: 1 in, 3 out]
            n170 = property on="Filename" class="Str"(error in=w471, "Value"=w463) -> (error out=w470:errorcluster)  [unwired: 1 in, 1 out]
          }
          frame "GUI Write - Scale Factor and Unit" {
            # "Assume they ALL have the same unit"
            n171 = call "Get Time Data Obj.vi"("reference in"=w492, "error in (no error)"=w491) -> ("Time data ref"=w485:refnum<class "GSwFormDSP.lvclass">, "error out"=w483:errorcluster)  [unwired: 15 in, 1 out]
            n172 = call-dynamic "Get - Names and Units.vi"("reference in"=w485, "error in (no error)"=w483) -> ("Signal Units"=w481:string[], "reference out"=w484:refnum<class "GSwFormDSP.lvclass">, "error out"=w482:errorcluster)  [unwired: 13 in, 2 out]
            n173 = call-dynamic "Math - Signals Statistics.vi"("reference in"=w484, "error in (no error)"=w482) -> ("Min's"=w487:dbl[], "Max's"=w488:dbl[], "error out"=w486:errorcluster)  [unwired: 10 in, 5 out]
            n174 = Build Array (concatenate)(w488, w487) -> (w489:dbl[])
            n175 = Index Array(array=w481) -> (element=w479:string)  [unwired: 1 in]
            n176 = Absolute Value(x=w489) -> (abs(x)=w490:dbl[])
            n177 = Array Max & Min(array=w490) -> (max value=w477:dbl)  [unwired: 3 out]
            n178 = property on="Scale Factor" class="DigNum (strict)"(error in=w486, "Value"=w477, "Minimum"=w477) -> (error out=w478:errorcluster)  [unwired: 1 in, 1 out]
            n179 = property on="Unit" class="Str"(error in=w478, "Value"=w479) -> (error out=w480:errorcluster)  [unwired: 1 in, 1 out]
          }
          frame "Refresh unit-factor-suffix controls" {
            n180 = case shown="\"No Change\", Default" "Unit Option" {
              tunnel: [T4."Enabled" ("Disabled") T4."Disabled and Grayed Out" ("Disabled")] -> w499
              tunnel: [w511 w513] -> w497
              tunnel: "Scale Factor" -> [w511 w519]
              tunnel: "Unit" -> [w507 _]
              tunnel: [w509 w521] -> w504
              tunnel: [w506 "_dB"] -> w503
              frame "No Change", Default {
                n181 = Number To Exponential String(number=w511, precision (6)=i16 2) -> (E-format string=w509:string)  [unwired: 2 in]
                n182 = Concatenate Strings("_" ("string"), w507) -> (w506:string)
              }
              frame "dB (Ref 20e-6 EU)" {
                w516 = 20.0 ("y")
                w514 = 2e-05 ("y")
                n183 = Divide(x=w519, y=w514) -> (x/y=w525:dbl)
                n184 = Logarithm Base 10(1:w525) -> (0:w524:dbl)
                n185 = Multiply(x=w524, y=w516) -> (x*y=w523:dbl)
                n186 = Round Toward +Infinity(x=w523) -> (ceil(x): smallest int >= x=w517:dbl)
                n187 = To Long Integer(number=w517) -> (32bit integer=w522:i32)
                n188 = Number To Decimal String(number=w522) -> (decimal integer string=w521:string)  [unwired: 1 in]
                n189 = Divide(x=w517, y=w516) -> (x/y=w518:dbl)
                n190 = Power Of 10(x=w518) -> (10^x=w515:dbl)
                n191 = Multiply(x=w514, y=w515) -> (x*y=w513:dbl)
              }
            }
            n192 = property on="Unit" class="Str"(error in=w493, "DisabledEnum"=w499) -> (error out=w498:errorcluster)  [unwired: 1 in, 1 out]
            n193 = property on="Scale Factor" class="DigNum (strict)"(error in=w498, "Value"=w497) -> (error out=w494:errorcluster)  [unwired: 1 in, 1 out]
            n194 = Concatenate Strings("_scale" ("string"), w504, w503) -> (w496:string)
            n195 = property on="Suffix" class="Str"(error in=w494, "Value"=w496) -> (error out=w495:errorcluster)  [unwired: 1 in, 1 out]
          }
        }
      }
      frame "FP" {
        n196 = case shown="\"Refresh\"" w527 {
          selector: w527 -> [w533 _ _]
          tunnel: w530 -> [_ w540 w552]
          tunnel: w529 -> [w532 w539 w551]
          tunnel: [w532 w536 w550] -> w528
          frame "", Default {
            n197 = Concatenate Strings("The following FP is unrecognized:\n", w533) -> (w534:string)
            n198 = One Button Dialog(message=w534) -> ()  [unwired: 1 in, 1 out]
          }
          frame "Open" {
            n199 = call-dynamic "Get VI Ref.vi"("reference in"=w540, "error in (no error)"=w539) -> ("GUI VI Ref"=w537:refnum<vi>, "error out"=w538:errorcluster)  [unwired: 14 in, 2 out]
            n200 = property class="VI"(reference=w537, error in=w538) -> (reference out=w542:refnum<vi>, error out=w543:errorcluster, "Front Panel.Open"=w541:bool)
            n201 = case shown="False" w541 {
              tunnel: [w546 w549] -> w536
              tunnel: w543 -> [w545 w549]
              tunnel: w542 -> [w544 _]
              frame False {
                n202 = invoke class="VI" method="FP.Open"(reference=w544, error in=w545, "Activate"=TRUE, "State"=T5."Standard") -> (error out=w546:errorcluster)  [unwired: 1 in, 4 out]
              }
              frame True {
              }
            }
          }
          frame "Refresh" {
            n203 = call "Get Time Data.vi"("reference in"=w552, "error in (no error)"=w551) -> ("wForms"=→"Time Data - READ":waveform(dbl)[], "error out"=w550:errorcluster)  [unwired: 14 in, 2 out]
          }
        }
      }
      frame "---- GUI Functions ----" {
      }
      frame "GUI: Initialize Ref" {
        n204 = case shown="\"GUI Write\"" w564 {
          tunnel: [T6."Default" ("Front Panel Window:Behavior") T6."Modal" ("Front Panel Window:Behavior")] -> w563
          frame "", Default {
          }
          frame "GUI Write" {
          }
        }
        n205 = control-ref of="GUI Reference"() -> (w565:refnum<vi>)
        n206 = call "Set VI Ref.vi"("reference in"=w571, "error in (no error)"=w568, "GUI VI Ref"=w565) -> ("reference out"=w570:refnum<class "WaveFile.lvclass">, "error out"=w566:errorcluster)  [unwired: 15 in]
        n207 = property class="VI"(reference=w565, error in=w566, "FP.Behavior"=w563) -> (error out=w562:errorcluster)  [unwired: 1 out]
        n208 = call "Set Close Panel (Yes or No).vi"("reference in"=w570, "error in (no error)"=w562) -> ("reference out"=w569:refnum<class "WaveFile.lvclass">, "error out"=w567:errorcluster)  [unwired: 16 in]
        n209 = call "Set Message Window Ref.vi"("reference in"=w569, "error in (no error)"=w567) -> ("reference out"=w560:refnum<class "WaveFile.lvclass">, "error out"=w561:errorcluster)  [unwired: 16 in]
        n210 = call "Get - Time Data OBJ State.vi"("reference in"=w560, "error in (no error)"=w561) -> ("New Time Data Obj?"=w559:bool, "reference out"=w558:refnum<class "WaveFile.lvclass">, "error out"=w557:errorcluster)  [unwired: 15 in]
        n211 = case shown="True" w559 {
          tunnel: w558 -> [_ w579]
          tunnel: w557 -> [w573 w578]
          tunnel: [w573 w574] -> w556
          frame False {
          }
          frame True {
            n212 = call "Get Time Data Obj.vi"("reference in"=w579, "error in (no error)"=w578) -> ("Time data ref"=w576:refnum<class "GSwFormDSP.lvclass">, "error out"=w575:errorcluster)  [unwired: 15 in, 1 out]
            n213 = call "Set - wForms.vi"("reference in"=w576, "error in (no error)"=w575, "Init wForms"=TRUE) -> ("error out"=w574:errorcluster)  [unwired: 15 in, 1 out]
          }
        }
      }
      frame "GUI: Exit" {
        n214 = call-dynamic "Get Message Window Ref.vi"("reference in"=w594, "error in (no error)"=w591) -> ("reference out"=w593:refnum<class "WaveFile.lvclass">, "Msg Win Ref"=w589:refnum<vi>, "error out"=w592:errorcluster)  [unwired: 15 in]
        n215 = call-dynamic "Get VI Ref.vi"("reference in"=w593, "error in (no error)"=w592) -> ("reference out"=w597:refnum<class "WaveFile.lvclass">, "GUI VI Ref"=w595:refnum<vi>, "error out"=w596:errorcluster)  [unwired: 14 in, 1 out]
        n216 = call-dynamic "Get Close Panel (Yes or No).vi"("reference in"=w597, "error in (no error)"=w596) -> ("Close Panel?"=w598:bool, "reference out"=w586:refnum<class "WaveFile.lvclass">, "error out"=w584:errorcluster)  [unwired: 15 in]
        n217 = call "Get - Time Data OBJ State.vi"("reference in"=w586, "error in (no error)"=w584) -> ("New Time Data Obj?"=w582:bool, "reference out"=w585:refnum<class "WaveFile.lvclass">, "error out"=w583:errorcluster)  [unwired: 15 in]
        n218 = call-dynamic "Destroy.vi"("reference in"=w585, "error in (no error)"=w583) -> ("error out"=w588:errorcluster)  [unwired: 16 in, 1 out]
        n219 = case shown="False" w582 {
          tunnel: w588 -> [w603 w605]
          tunnel: [w603 w604] -> w587
          frame False {
          }
          frame True {
            n220 = call <vilib>:"GarbageCollector.vi"("error in (no error)"=w605) -> ("error out"=w604:errorcluster)  [unwired: 16 in, 2 out]
          }
        }
        n221 = Close Reference(reference=w589, error in (no error)=w587) -> (error out=w601:errorcluster)
        n222 = case shown="True" w598 {
          tunnel: w601 -> [w607 w611]
          tunnel: [w607 w610] -> w599
          tunnel: [w606 w609] -> w600
          tunnel: w595 -> [w606 w608]
          frame False {
          }
          frame True {
            n223 = property class="VI"(reference=w608, error in=w611) -> (reference out=w613:refnum<vi>, error out=w612:errorcluster, "Front Panel.Open"=w614:bool)
            n224 = case shown="True" w614 {
              tunnel: [w616 w620] -> w610
              tunnel: w612 -> [w616 w619]
              tunnel: w613 -> [w615 w618]
              tunnel: [w615 w617] -> w609
              frame False {
              }
              frame True {
                n225 = invoke class="VI" method="FP.Close"(reference=w618, error in=w619) -> (reference out=w617:refnum<vi>, error out=w620:errorcluster)  [unwired: 1 in, 1 out]
              }
            }
          }
        }
        n226 = Close Reference(reference=w600, error in (no error)=w599) -> (error out=w590:errorcluster)
      }
      frame "SEND MSG" {
        n227 = call-dynamic "Get Message Window Ref.vi"("reference in"=w625, "error in (no error)"=w624) -> ("Msg Win Ref"=w621:refnum<vi>, "error out"=w623:errorcluster)  [unwired: 15 in, 1 out]
        n228 = property class="VI"(reference=w621, error in=w623) -> (reference out=w627:refnum<vi>, error out=w626:errorcluster, "Front Panel.Open"=w628:bool)
        n229 = case shown="False" w628 {
          tunnel: [w642 w646] -> w630
          tunnel: w626 -> [w637 w646]
          tunnel: w627 -> [w639 w645]
          tunnel: [w641 w645] -> w629
          frame False {
            w640 = FALSE ("Wait Until Done")
            n230 = invoke class="VI" method="Run VI"(reference=w639, error in=w637, "Wait until done"=w640, "Auto Dispose Ref"=w640) -> (reference out=w638:refnum<vi>, error out=w636:errorcluster)  [unwired: 1 in, 3 out]
            n231 = invoke class="VI" method="FP.Open"(reference=w638, error in=w636, "Activate"=TRUE, "State"=T5."Standard") -> (reference out=w641:refnum<vi>, error out=w642:errorcluster)  [unwired: 1 in, 3 out]
          }
          frame True {
          }
        }
        n232 = Concatenate Strings("\r\n", w634) -> (w633:string)
        n233 = invoke class="VI" method="Ctrl Val.Set"(reference=w629, error in=w630, "Control Name"="Message", "Value"=w633) -> (error out=w622:errorcluster)  [unwired: 1 in, 4 out]
      }
      frame "CLOSE MSG" {
        n234 = call-dynamic "Get Message Window Ref.vi"("reference in"=w650, "error in (no error)"=w651) -> ("Msg Win Ref"=w648:refnum<vi>, "error out"=w649:errorcluster)  [unwired: 15 in, 1 out]
        n235 = property class="VI"(reference=w648, error in=w649) -> (reference out=w655:refnum<vi>, error out=w656:errorcluster, "Front Panel.Open"=w654:bool)
        n236 = case shown="True" w654 {
          tunnel: [w659 w663] -> w653
          tunnel: w656 -> [w659 w662]
          tunnel: w655 -> [w658 w661]
          tunnel: [w658 w660] -> w652
          frame False {
          }
          frame True {
            n237 = invoke class="VI" method="FP.Close"(reference=w661, error in=w662) -> (reference out=w660:refnum<vi>, error out=w663:errorcluster)  [unwired: 1 in, 1 out]
          }
        }
        n238 = invoke class="VI" method="Abort VI"(reference=w652, error in=w653) -> (error out=w647:errorcluster)  [unwired: 1 in, 2 out]
      }
      frame "---- Miscelleneous ----" {
      }
      frame "unknown", Default {
        n239 = Concatenate Strings("The following state is unrecognized?\n", w668) -> (w667:string)
        n240 = One Button Dialog(message=w667) -> ()  [unwired: 1 in, 1 out]
      }
      frame "Error" {
        n241 = call <vilib>:"General Error Handler.vi"("error in (no error)"=w671) -> ()  [unwired: 10 in, 5 out]
      }
      frame "Next" {
        # "This is an empty case used so the queue does NOT stop if there is an empty string between two valid states!"
      }
      frame "Quit" {
        # "This is the case used to simply exit when this GUI is used as a SubVI!"
        n242 = call-dynamic "Destroy.vi"("reference in"=w677, "error in (no error)"=w676) -> ("error out"=w678:errorcluster)  [unwired: 16 in, 1 out]
      }
    }
    "State Index" <- w17
  }
  "error out" <- w2
  "SubVI Time Data DUP" <- "Time Data IN"
